vi "Send Refresh Rooms Status.vi"(7 "Message Priority (Normal)":T2=enum."Normal", 8 "error in (no error)":errorcluster, 10 "Room Details":T1[](array[typedef]), 11 "Message Enqueuer":refnum<class "Message Enqueuer.lvclass">) -> (0 "error out":errorcluster, 3 "Message Enqueuer out":refnum<class "Message Enqueuer.lvclass">)   [LabVIEW 2023, in "Rooms Manager UI.lvlib" / "Refresh Rooms Status Msg.lvclass"]
doc: "This VI sends the message to an actor."
uses:
  Refresh Rooms Status Msg.lvclass
  <vilib>/ActorFramework/Message Enqueuer/Message Enqueuer.lvclass
  <vilib>/ActorFramework/Message Enqueuer/Message Priority.ctl
  Rooms Manager UI/Room Status.ctl
  Refresh Rooms Status Msg.lvclass/Refresh Rooms Status Msg.ctl
  <vilib>/ActorFramework/Message Enqueuer/Message Enqueuer.lvclass/Message Enqueuer.ctl
  <vilib>/ActorFramework/Message Priority Queue/Priority Enqueue.vi
  Rooms Manager UI/Rooms Manager UI.lvclass
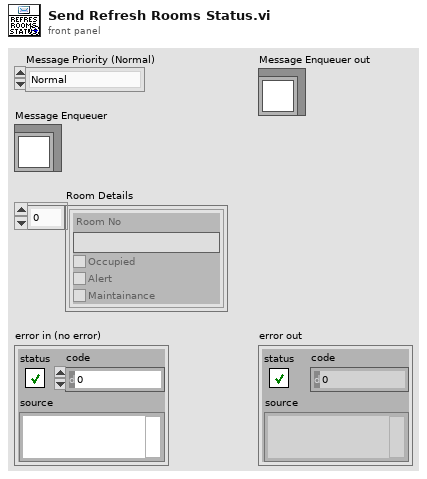
[diagram p1: front panel]
types:
  T1 = typedef "Rooms Manager UI.lvlib/Rooms Manager UI.lvclass/Room Status.ctl" = cluster{"Room No":string, "Occupied":bool, "Alert":bool, "Maintainance":bool}
  T2 = typedef "Actor Framework.lvlib/Message Enqueuer.lvclass/Message Priority.ctl" = enum16{"Low", "Normal", "High"}
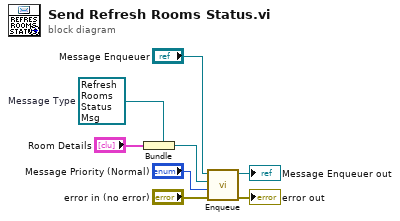
[diagram p0: block diagram]
diagram:
  w5 = refnum<class "Refresh Rooms Status Msg.lvclass"> refnum  # Message Type
  n1 = Bundle(cluster=w5, "Room Details") -> (w4:refnum<class "Refresh Rooms Status Msg.lvclass">)
  n2 = call <vilib>:"Enqueue.vi"("error in (no error)"="error in (no error)", "Message Priority (Normal)"="Message Priority (Normal)", "Message"=w4, "Message Enqueuer in"="Message Enqueuer") -> ("error out"=→"error out":errorcluster, "Message Enqueuer out"=→"Message Enqueuer out":refnum<class "Message Enqueuer.lvclass">)  [unwired: 6 in]
